vi "FrequencyAnalysis.vi"(0 "System no.":i32=1 min=1 step=1, 1 "Analog Input Channel":u32=1, 5 "error in":errorcluster) -> (19 "error out":errorcluster)   [LabVIEW 2020]
doc: "This VI allows the user to analyze oscillations on the optical path.\nFor more information, please refer to the documentation of this sample application."
uses:
  <vilib>/Utility/miscctls.llb/LVCursorListTypeDef.ctl
  C:/ProgramData/PI/LabVIEW/Low Level/GeneralCommands/Global2 (Array).vi
  <vilib>/Analysis/NI_AALPro.lvlib
panel:
  out "Sample Time":dbl format="%.10f"
  in  "Read":bool
  out "Curser X position:":dbl
  in  "Raw Data":bool
  out "2DArray":dbl[][](array[numeric])
  in  "Impulse":bool
  in  "Servo":bool=TRUE
  in  "Impulse size":dbl=1.0
  in  "Axis":u16(ring) items=["1", "2", "3", "4", "5", "6", "7", "8", "9", "10", "11", "12"]
  in  "# of data points":i32=8192
  in  "Record Rate - # cycles":i32=1
  in  "FFT":bool
  out "XY Graph":cluster{dbl[], "Data":dbl[]}(graph)
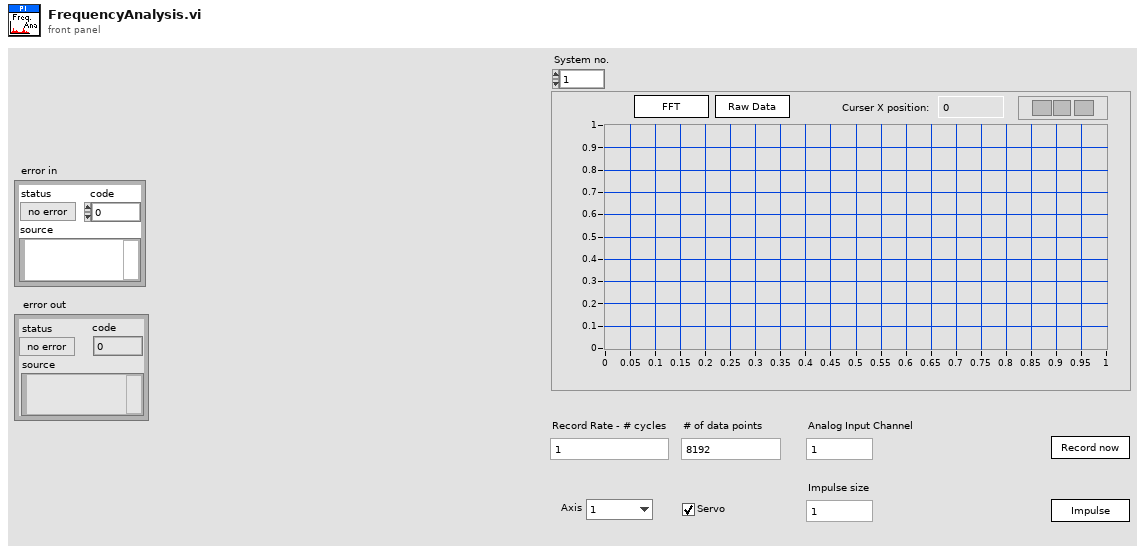
[diagram p1: front panel]
types:
  T1 = typedef "LVCursorListTypeDef.ctl" = cluster{"Name":string, "Color":u32, "Style":u8, "Point Style":u8, "Name Visible":bool, "Allow Drag":bool, "Cursor Mode":u32, "Plot":i32, "Index":i32, "Position":cluster{"X":dbl, "Y":dbl}, "X Scale":u32, "Y Scale":u32, "Watch Plots":i32[], "Watch All Plots":bool, "Plot Area":i32, "Label Offset":cluster{"X":dbl, "Y":dbl}}[]
  T2 = typedef "Controller names.ctl" = enum16{"None", "Analog", "C-702", "C-413", "C-414", "C-843", "C-843.PM", "C-844", "C-848", "C-865", "C-866", "C-867", "C-877", "C-880", "C-884", "C-885", "C-886", "C-887", "C-891", "E-135", "E-516", "E-517", "E-518", "E-709", "E-710", "E-712", "E-725", "E-727", "E-753", "E-754", "E-755", "E-761", "E-816", "E-861", "E-870", "E-871", "E-872", "E-873", "E-874", "F-206", "HydraPollux", "M-840", "M-850", "M-8X0", "Mercury", "Mercury_GCS", "PI_GCS2"}
  T3 = cluster{"Conn. axes":string[], "Controller name":T2}[]
  T4 = cluster{"Conn. axes":string[], "Controller name":T2}
  T5 = typedef "LVPoint32TypeDef.ctl" = cluster{"Horizontal":i32, "Vertical":i32}
  T6 = typedef "LVRectTypeDef.ctl" = cluster{"Left":i16, "Top":i16, "Right":i16, "Bottom":i16}
  T7 = cluster{"Name":string, "Color":u32, "Style":u8, "Point Style":u8, "Name Visible":bool, "Allow Drag":bool, "Cursor Mode":u32, "Plot":i32, "Index":i32, "Position":cluster{"X":dbl, "Y":dbl}, "X Scale":u32, "Y Scale":u32, "Watch Plots":i32[], "Watch All Plots":bool, "Plot Area":i32, "Label Offset":cluster{"X":dbl, "Y":dbl}}
  T8 = cluster{"Name":string, "Color":u32, "Style":u8, "Point Style":u8, "Name Visible":bool, "Allow Drag":bool, "Cursor Mode":u32, "Plot":i32, "Index":i32, "Position":cluster{"X":dbl, "Y":dbl}, "X Scale":u32, "Y Scale":u32, "Watch Plots":i32[], "Watch All Plots":bool, "Plot Area":i32, "Label Offset":cluster{"X":dbl, "Y":dbl}}[]
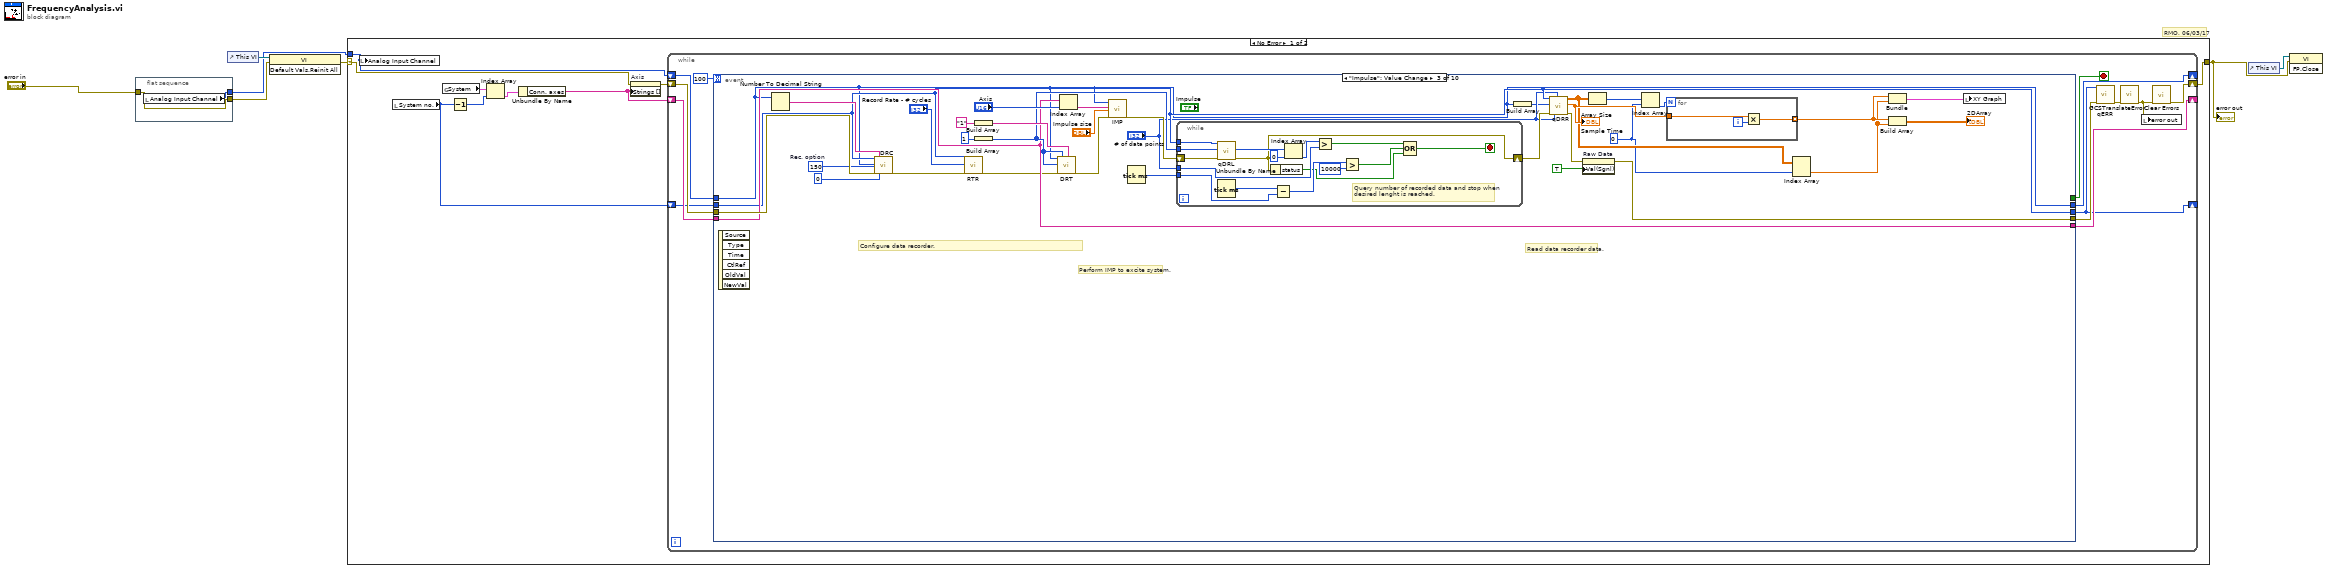
[diagram p0: block diagram]
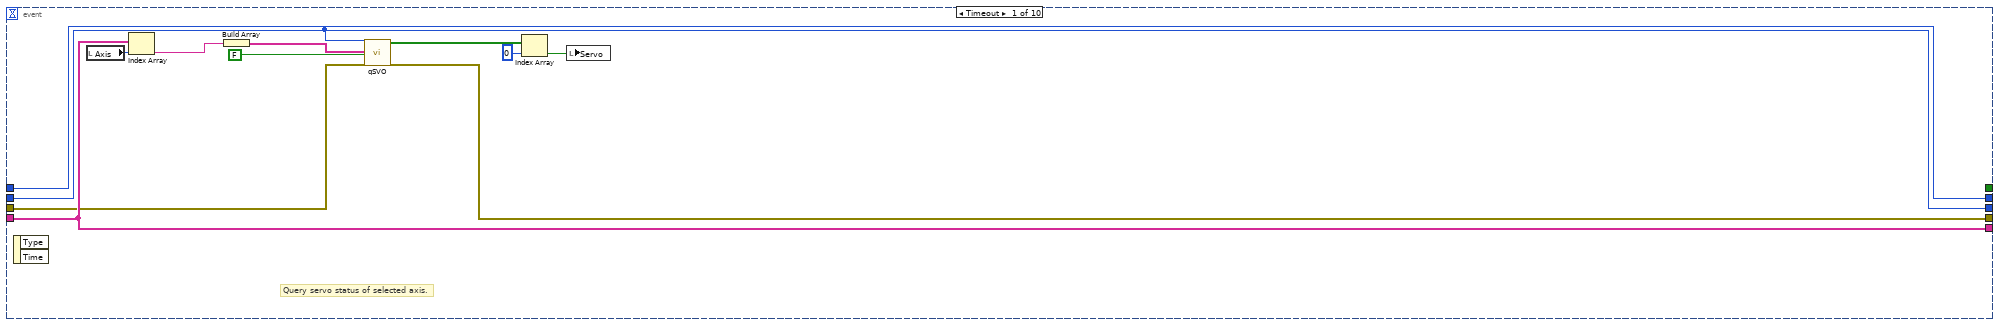
[diagram p2: hidden frame]
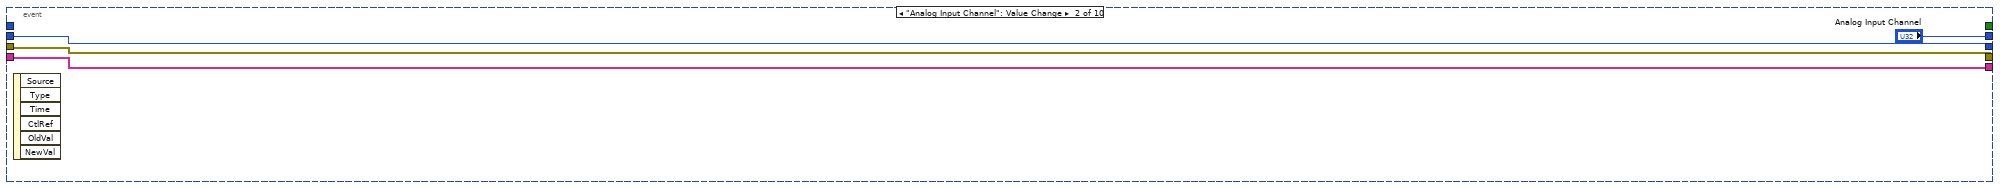
[diagram p3: hidden frame]
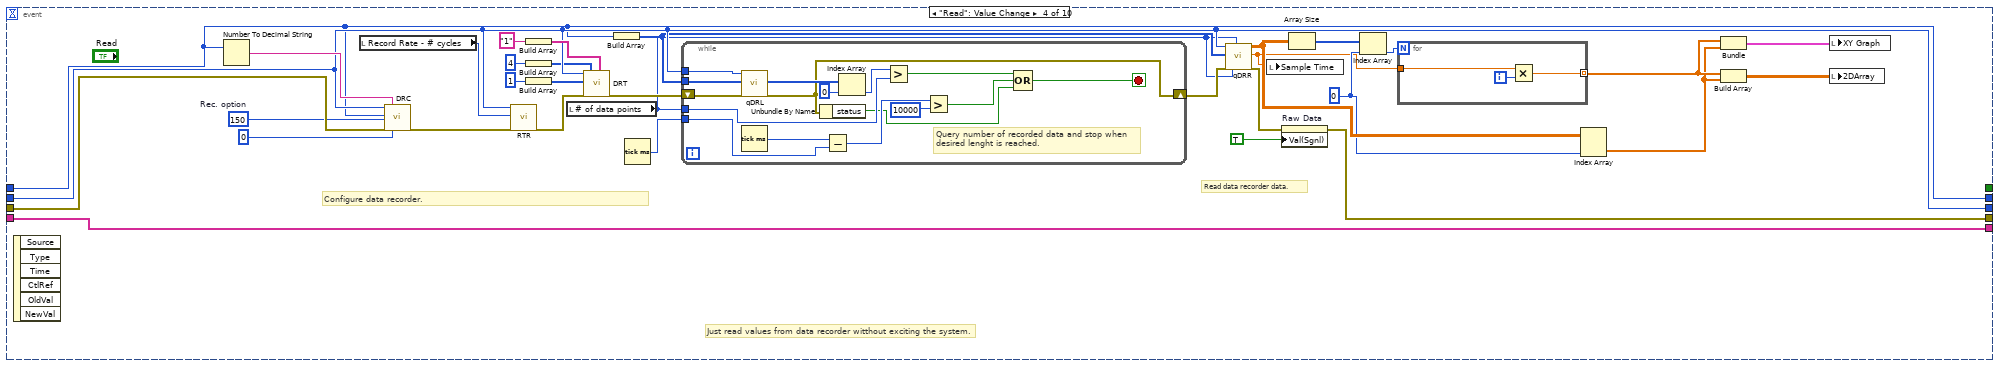
[diagram p4: hidden frame]
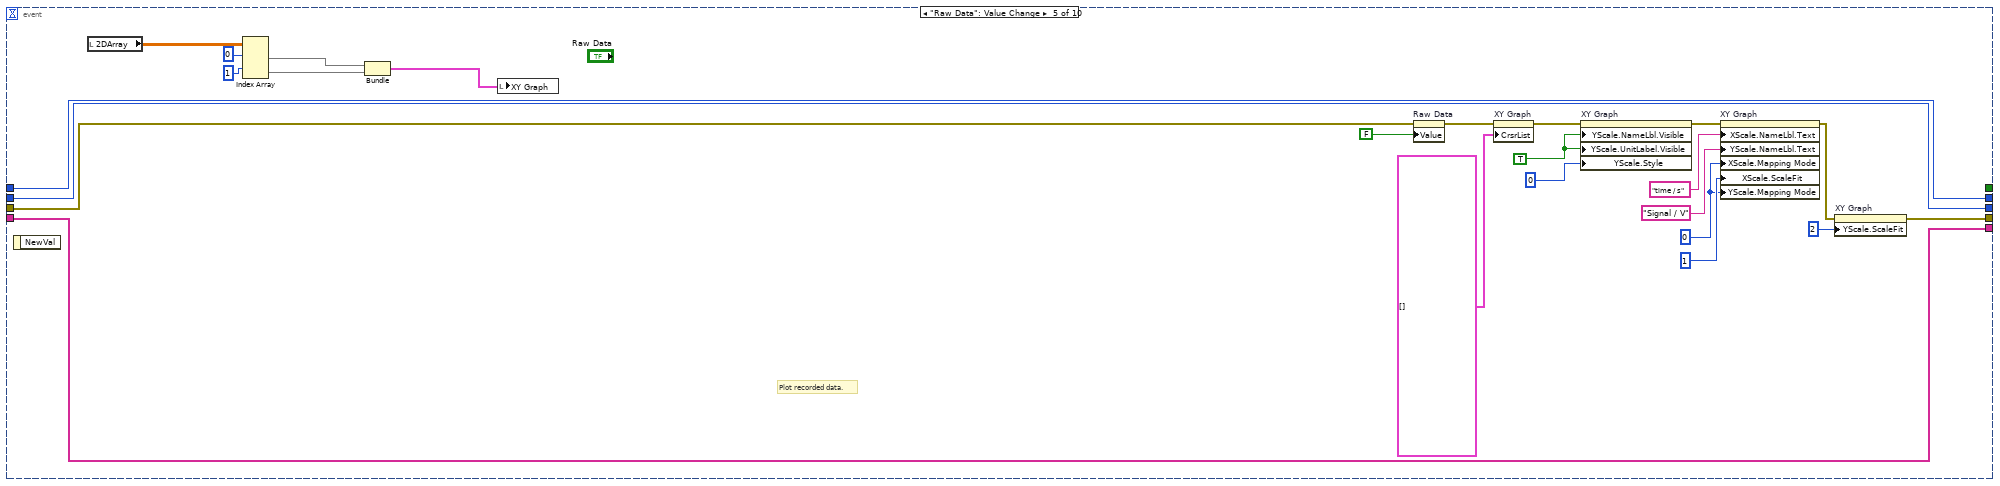
[diagram p5: hidden frame]
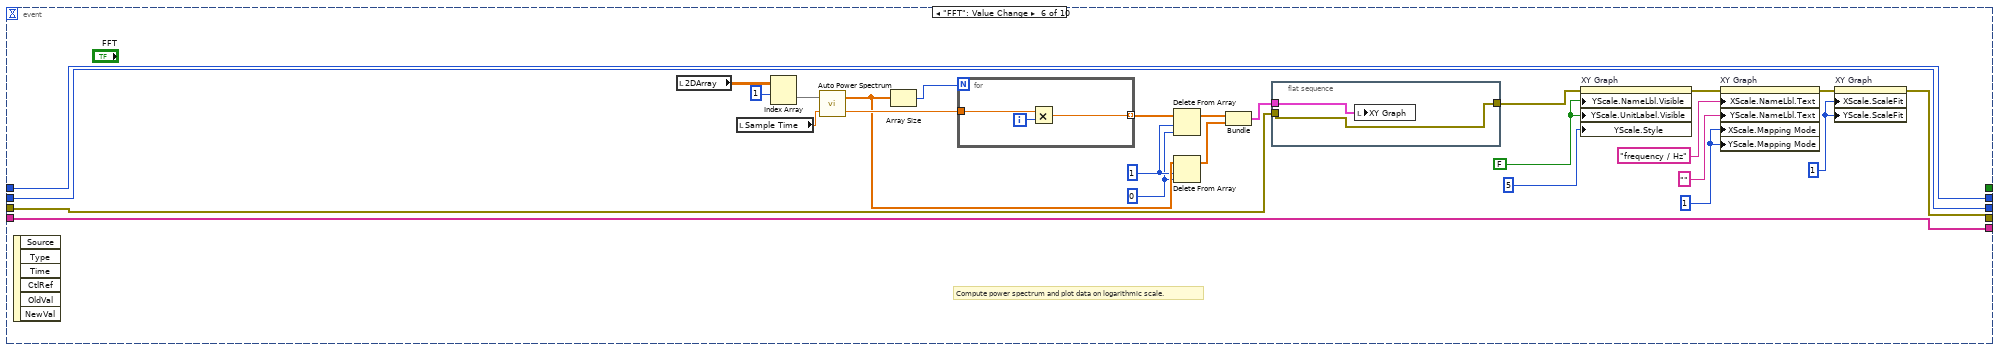
[diagram p6: hidden frame]
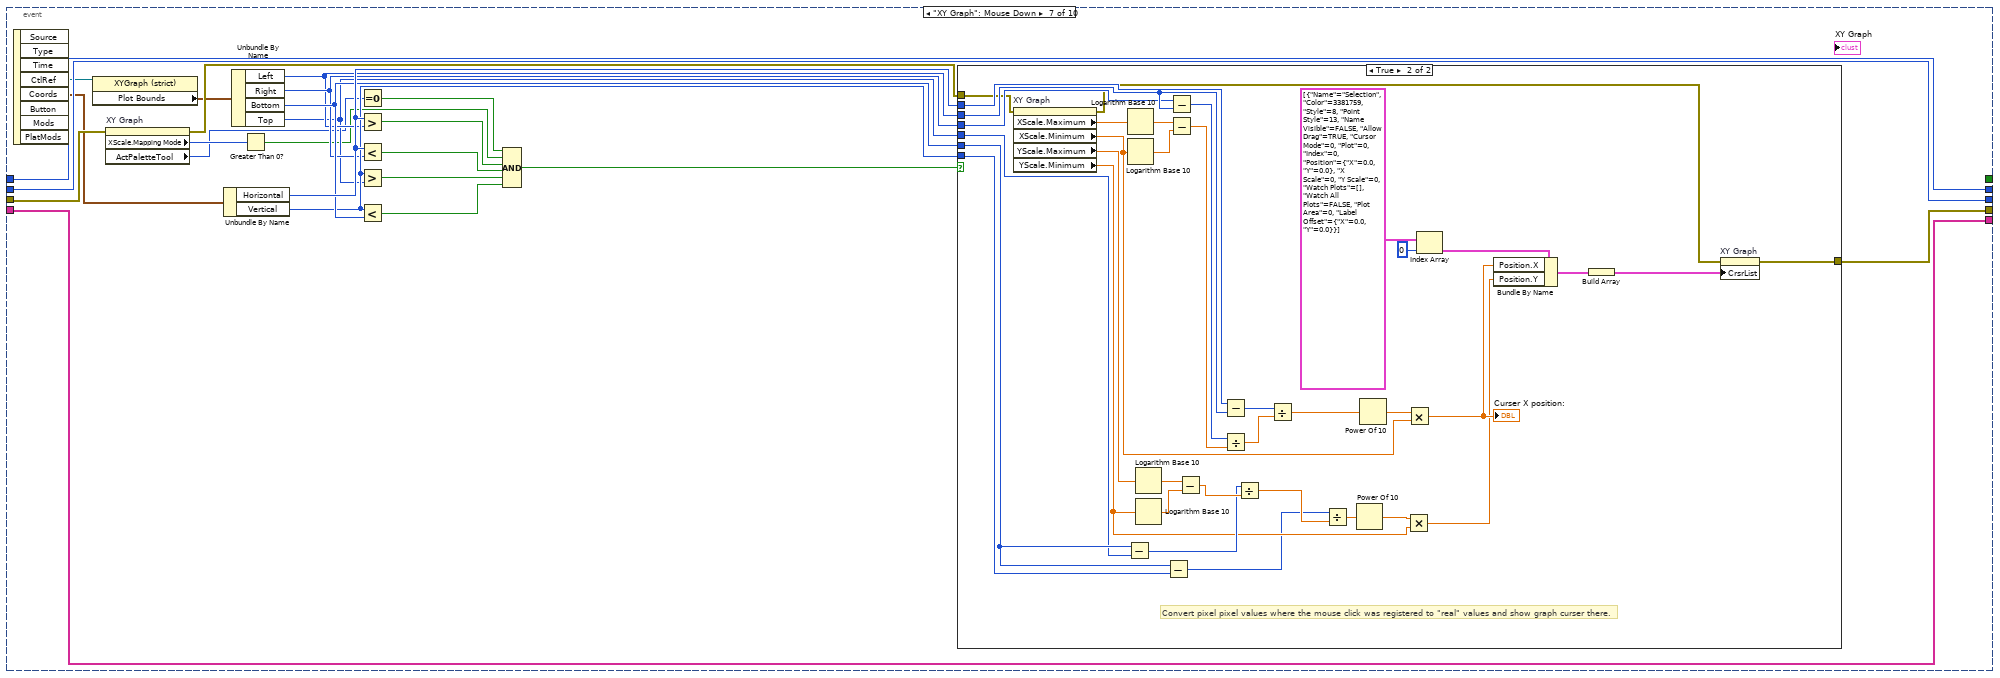
[diagram p7: hidden frame]
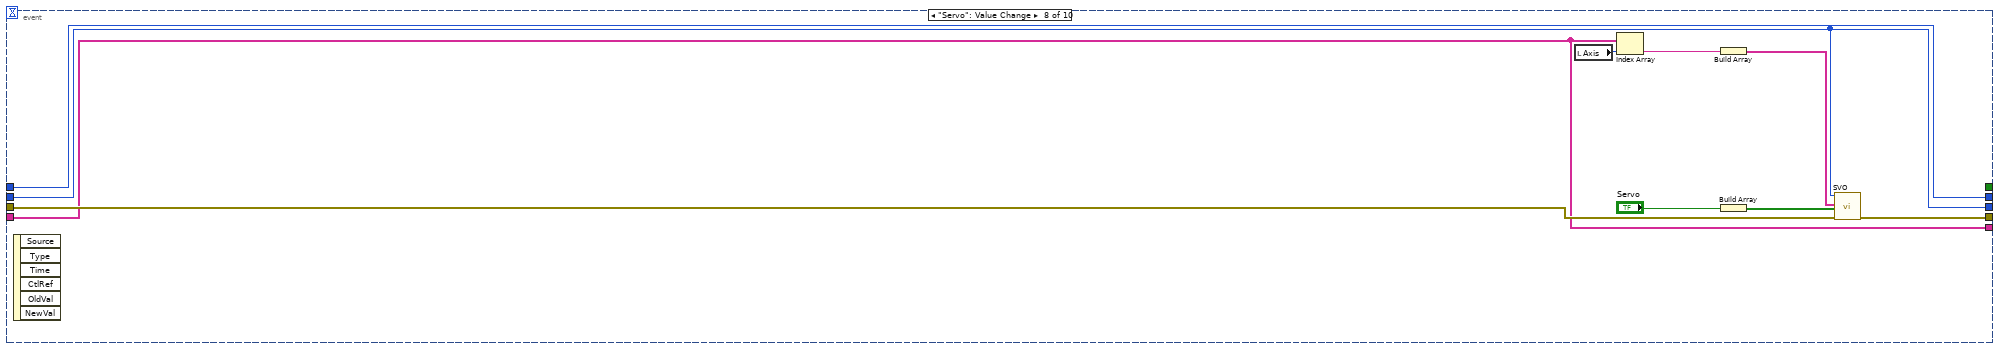
[diagram p9: hidden frame]
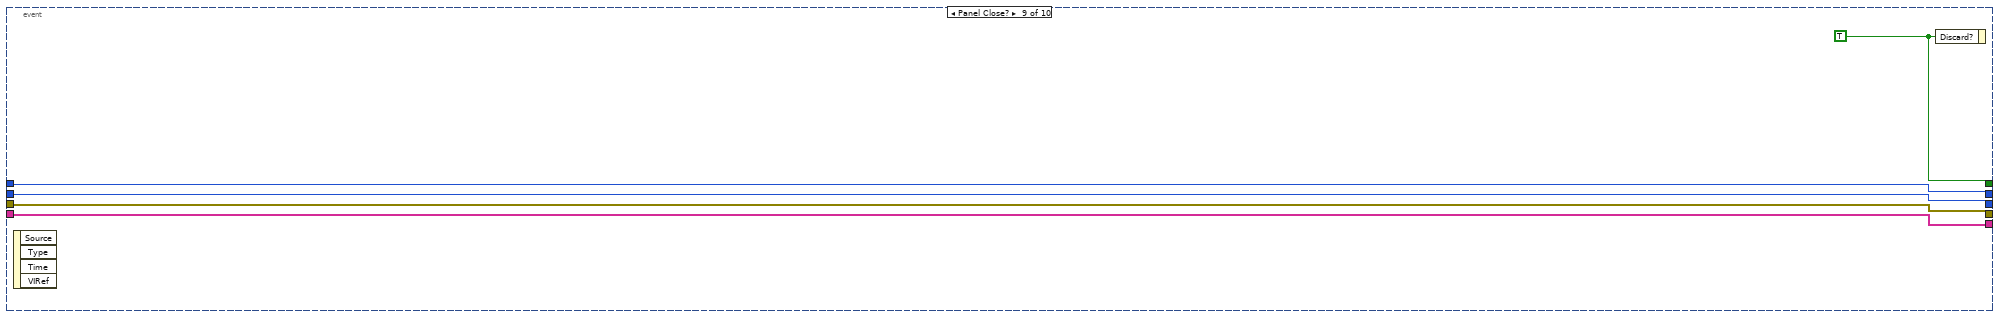
[diagram p10: hidden frame]
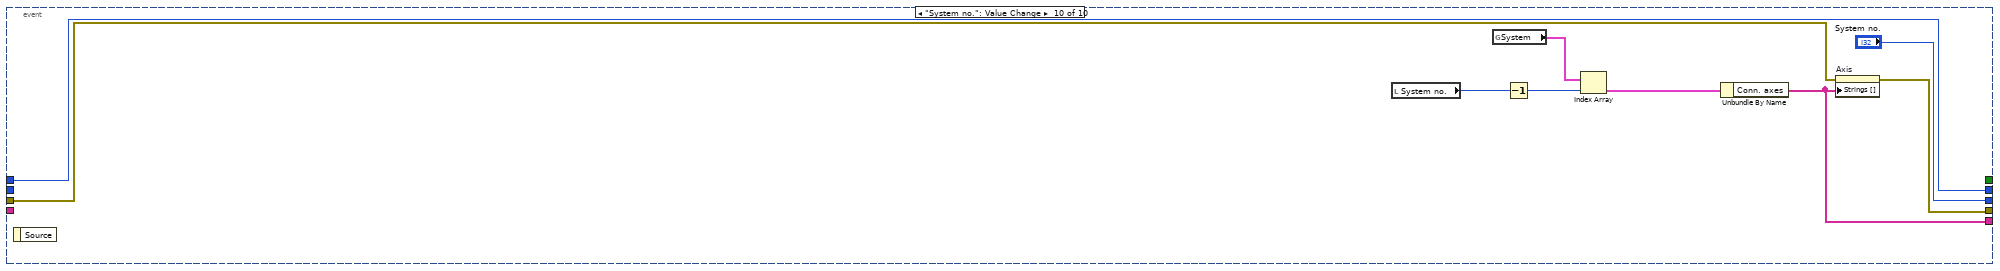
[diagram p11: hidden frame]
diagram:
  # "RMO, 06/03/17"
  n1 = flat-sequence {
    tunnel: "error in" -> [w9]
    tunnel: [w9] -> w4
    tunnel: [w8] -> w3
    frame #0 {
      n2 = local read "Analog Input Channel"() -> (w8:u32)
    }
  }
  n3 = control-ref of="This VI"() -> (w6:refnum<vi>)
  n4 = invoke class="VI" method="Default Vals.Reinit All"(reference=w6, error in=w4) -> (error out=w5:errorcluster)  [unwired: 1 in, 2 out]
  n5 = case shown="No Error" w5 {
    selector: w5 -> [w13 w295]
    tunnel: [w15 w295] -> w7
    tunnel: w3 -> [w10 _]
    frame No Error {
      n6 = local write "Analog Input Channel"(w10) -> ()
      n7 = local read "System no."() -> (w14:i32)
      n8 = global read "Global2 (Array).vi" "System"() -> (w18:T3)
      n9 = Decrement(x=w14) -> (x-1=w17:i32)
      n10 = Index Array(array=w18, index=w17) -> (element=w16:T4)
      n11 = Unbundle By Name(w16) -> ("Conn. axes"=w11:string[])
      n12 = property on="Axis" class="Ring (strict)"(error in=w13, "Strings []"=w11) -> (error out=w12:errorcluster)  [unwired: 1 in, 1 out]
      n13 = while {
        shift-right: [w24] -> w15
        shift-left: w12 -> [w30]
        shift-right: [w22] -> _
        shift-left: w11 -> [w31]
        shift-right: [w21] -> _
        shift-left: w14 -> [w25]
        shift-right: [w20] -> _
        shift-left: w10 -> [w19]
        stop <- w29 stop-if-true
        n14 = event shown="[2] \"Impulse\": Value Change" {
          selector: _ -> [_ _ _ _ _ _ _ _ _ _]
          dyn-events: _ -> [_ _ _ _ _ _ _ _ _ _]
          timeout: 100 -> [_ _ _ _ _ _ _ _ _ _]
          tunnel: w31 -> [w36 w45 w64 w122 w175 w202 w232 w274 w284 _]
          tunnel: w30 -> [w32 w44 w77 w130 w161 w183 w233 w280 w283 w290]
          tunnel: [w41 w44 w56 w115 w155 w188 w215 w273 w283 w289] -> w27
          tunnel: [_ _ _ _ _ _ _ _ w285 _] -> w29
          tunnel: w25 -> [w42 w46 w63 w121 w176 w203 w231 w272 w282 _]
          tunnel: [w36 w45 w64 w122 w175 w202 w232 w274 w284 w288] -> w22
          tunnel: [w42 w46 w63 w121 w176 w203 w231 w272 w282 "System no."] -> w21
          tunnel: [w43 "Analog Input Channel" w50 w106 w177 w204 w230 w271 w281 w287] -> w20
          tunnel: w19 -> [w43 _ w50 w106 w177 w204 w230 w271 w281 w287]
          event Timeout {
            # "Query servo status of selected axis."
            n15 = event-data() -> ()  [unwired: 3 out]
            n16 = local read "Axis"() -> (w33:u16)
            n17 = Index Array(array=w36, index=w33) -> (element=w35:string)
            n18 = Build Array(w35) -> (w34:string[])
            n19 = call "qSVO.vi"("System no."=w42, "Axes to query"=w34, "All axes?"=FALSE, "error in"=w32) -> ("Servo status?"=w40:bool[], "error out"=w41:errorcluster)  [unwired: 1 in, 13 out]
            n20 = Index Array(array=w40, index=0) -> (element=w38:bool)
            n21 = local write "Servo"(w38) -> ()
          }
          event "Analog Input Channel": Value Change {
            n22 = event-data() -> ()  [unwired: 7 out]
          }
          event "Impulse": Value Change {
            w48 = 150  # Rec. option
            w62 = 0 ("index")
            # "Read data recorder data."
            # "Perform IMP to excite system."
            # "Configure data recorder."
            n23 = event-data() -> ()  [unwired: 7 out]
            n24 = Number To Decimal String(number=w50) -> (decimal integer string=w76:string)  [unwired: 1 out]
            n25 = call "DRC.vi"("System no."=w63, "Rec. table"=w50, "Rec. option"=w48, "error in"=w77, "Source ID"=w76, "Trigger option"=0) -> ("error out"=w52:errorcluster)  [unwired: 13 out]
            n26 = call "RTR.vi"("System no."=w63, "Table rate"="Record Rate - # cycles", "error in"=w52) -> ("error out"=w53:errorcluster)  [unwired: 16 out]
            n27 = Build Array("1") -> (w80:string[])
            n28 = Build Array(1) -> (w69:i32[])
            n29 = call "DRT.vi"("System no."=w63, "DataRecorderTable"=w69, "error in"=w53, "Trigger source"=w69, "Value"=w80) -> ("error out"=w54:errorcluster)  [unwired: 14 out]
            n30 = Index Array(array=w64, index="Axis") -> (element=w74:string)
            n31 = call "IMP.vi"("System no."=w63, "Axis to command"=w74, "Impulse size"="Impulse size", "error in"=w54) -> ("error out"=w71:errorcluster)  [unwired: 1 in, 14 out]
            n32 = Tick Count (ms)() -> (millisecond timer value=w72:u32)
            n33 = while {
              tunnel: w63 -> [w101]
              tunnel: w69 -> [w100]
              tunnel: "# of data points" -> [w96]
              tunnel: w72 -> [w94]
              shift-right: [w86] -> w70
              shift-left: w71 -> [w91]
              stop <- w87 stop-if-true
              # "Query number of recorded data and stop when desired lenght is reached."
              n34 = call "qDRL.vi"("System no."=w101, "Rec. table to query"=w100, "error in"=w91) -> ("No. of rec. values"=w99:i32[], "error out"=w86:errorcluster)  [unwired: 1 in, 14 out]
              n35 = Tick Count (ms)() -> (millisecond timer value=w95:u32)
              n36 = Unbundle By Name(w86) -> ("status"=w88:bool)
              n37 = Subtract(x=w95, y=w94) -> (x-y=w93:u32)
              n38 = Index Array(array=w99, index=0) -> (element=w97:i32)
              n39 = Greater?(x=w97, y=w96) -> (0:w90:bool)
              n40 = Greater?(x=w93, y=u32 10000) -> (0:w89:bool)
              n41 = Compound Arithmetic op=OR(w90, w89, w88) -> (w87:bool)
            }
            n42 = Build Array(w50) -> (w49:u32[])
            n43 = call "qDRR.vi"("System no."=w63, "Rec. table IDs"=w49, "error in"=w70, "N"="# of data points", "Nmax"="# of data points") -> ("Data"=w65:dbl[][], "Sample Time"=w66:dbl, "error out"=w57:errorcluster)  [unwired: 3 in, 9 out]
            "Sample Time" <- w66
            n44 = property on="Raw Data" class="Bool (strict)"(error in=w57, "Val(Sgnl)"=TRUE) -> (error out=w56:errorcluster)  [unwired: 1 in, 1 out]
            n45 = Array Size(array=w65) -> (size(s)=w68:i32[])
            n46 = Index Array(array=w68, index=w62) -> (element=w67:i32)
            n47 = for {
              N: w67 -> [_]
              tunnel: w66 -> [w85]
              tunnel: [w84] -> w61 mode=indexing
              i -> [w83]
              n48 = Multiply(x=w85, y=w83) -> (x*y=w84:dbl)
            }
            n49 = Index Array(array=w65, index (col)=w62) -> (element=w60:dbl[])  [unwired: 1 in]
            n50 = Bundle(w61, "Data"=w60) -> (w58:cluster{dbl[], "Data":dbl[]})  [unwired: 1 out]
            n51 = Build Array(w61, w60) -> (→"2DArray":dbl[][])
            n52 = local write "XY Graph"(w58) -> ()
          }
          event "Read": Value Change {
            w102 = 150  # Rec. option
            w120 = 0 ("index")
            # "Just read values from data recorder witthout exciting the system."
            # "Read data recorder data."
            # "Configure data recorder."
            n53 = event-data() -> ()  [unwired: 7 out]
            n54 = Number To Decimal String(number=w106) -> (decimal integer string=w129:string)  [unwired: 1 out]
            n55 = local read "Record Rate - # cycles"() -> (w113:i32)
            n56 = call "DRC.vi"("System no."=w121, "Rec. table"=w106, "Rec. option"=w102, "error in"=w130, "Source ID"=w129, "Trigger option"=0) -> ("error out"=w109:errorcluster)  [unwired: 13 out]
            n57 = call "RTR.vi"("System no."=w121, "Table rate"=w113, "error in"=w109) -> ("error out"=w108:errorcluster)  [unwired: 16 out]
            n58 = Build Array("1") -> (w132:string[])
            n59 = Build Array(4) -> (w111:i32[])
            n60 = Build Array(1) -> (w126:i32[])
            n61 = local read "# of data points"() -> (w103:i32)
            n62 = call "DRT.vi"("System no."=w121, "DataRecorderTable"=w126, "error in"=w108, "Trigger source"=w111, "Value"=w132) -> ("error out"=w107:errorcluster)  [unwired: 14 out]
            n63 = Build Array(w106) -> (w105:u32[])
            n64 = Tick Count (ms)() -> (millisecond timer value=w128:u32)
            n65 = while {
              tunnel: w121 -> [w153]
              tunnel: w105 -> [w152]
              tunnel: w103 -> [w148]
              tunnel: w128 -> [w146]
              shift-right: [w138] -> w127
              shift-left: w107 -> [w143]
              stop <- w139 stop-if-true
              # "Query number of recorded data and stop when desired lenght is reached."
              n66 = call "qDRL.vi"("System no."=w153, "Rec. table to query"=w152, "error in"=w143) -> ("No. of rec. values"=w151:i32[], "error out"=w138:errorcluster)  [unwired: 1 in, 14 out]
              n67 = Tick Count (ms)() -> (millisecond timer value=w147:u32)
              n68 = Unbundle By Name(w138) -> ("status"=w140:bool)
              n69 = Subtract(x=w147, y=w146) -> (x-y=w145:u32)
              n70 = Index Array(array=w151, index=0) -> (element=w149:i32)
              n71 = Greater?(x=w149, y=w148) -> (0:w142:bool)
              n72 = Greater?(x=w145, y=u32 10000) -> (0:w141:bool)
              n73 = Compound Arithmetic op=OR(w142, w141, w140) -> (w139:bool)
            }
            n74 = call "qDRR.vi"("System no."=w121, "Rec. table IDs"=w105, "error in"=w127, "N"=w103, "Nmax"=w103) -> ("Data"=w123:dbl[][], "Sample Time"=w104:dbl, "error out"=w116:errorcluster)  [unwired: 3 in, 9 out]
            n75 = local write "Sample Time"(w104) -> ()
            n76 = property on="Raw Data" class="Bool (strict)"(error in=w116, "Val(Sgnl)"=TRUE) -> (error out=w115:errorcluster)  [unwired: 1 in, 1 out]
            n77 = Array Size(array=w123) -> (size(s)=w125:i32[])
            n78 = Index Array(array=w125, index=w120) -> (element=w124:i32)
            n79 = for {
              N: w124 -> [_]
              tunnel: w104 -> [w137]
              tunnel: [w136] -> w119 mode=indexing
              i -> [w135]
              n80 = Multiply(x=w137, y=w135) -> (x*y=w136:dbl)
            }
            n81 = Index Array(array=w123, index (col)=w120) -> (element=w118:dbl[])  [unwired: 1 in]
            n82 = Bundle(w119, "Data"=w118) -> (w117:cluster{dbl[], "Data":dbl[]})  [unwired: 1 out]
            n83 = Build Array(w119, w118) -> (w112:dbl[][])
            n84 = local write "XY Graph"(w117) -> ()
            n85 = local write "2DArray"(w112) -> ()
          }
          event "Raw Data": Value Change {
            w157 = u8 0 ("X Scale.Mapping Mode")
            w165 = TRUE ("Y Scale.Name Label.Visible")
            # "Plot recorded data."
            n86 = event-data() -> ()  [unwired: 2 out]
            n87 = local read "2DArray"() -> (w172:dbl[][])
            n88 = Index Array(array=w172, index (row) #1=0 ("disabled index (col)"), index (row) #2=1 ("disabled index (col)")) -> (element #1=w171:dbl[], element #2=w170:dbl[])  [unwired: 2 in]
            n89 = Bundle("2DArray"=w171, "2DArray"=w170) -> (w169:cluster{"2DArray":dbl[], "2DArray":dbl[]})  [unwired: 1 out]
            n90 = local write "XY Graph"(w169) -> ()
            n91 = property on="Raw Data" class="Bool (strict)"(error in=w161, "Value"=FALSE) -> (error out=w160:errorcluster)  [unwired: 1 in, 1 out]
            n92 = property on="XY Graph" class="XYGraph (strict)"(error in=w160, "CrsrList"=T1 [] ("Cursor List")) -> (error out=w163:errorcluster)  [unwired: 1 in, 1 out]
            n93 = property on="XY Graph" class="XYGraph (strict)"(error in=w163, "YScale.NameLbl.Visible"=w165, "YScale.UnitLabel.Visible"=w165, "YScale.Style"=u8 0 ("Y Scale.Style")) -> (error out=w166:errorcluster)  [unwired: 1 in, 1 out]
            n94 = property on="XY Graph" class="XYGraph (strict)"(error in=w166, "XScale.NameLbl.Text"="time / s" ("X Scale.Name Label.Text"), "YScale.NameLbl.Text"="Signal / V" ("Y Scale.Name Label.Text"), "XScale.Mapping Mode"=w157, "XScale.ScaleFit"=1, "YScale.Mapping Mode"=w157) -> (error out=w156:errorcluster)  [unwired: 1 in, 1 out]
            n95 = property on="XY Graph" class="XYGraph (strict)"(error in=w156, "YScale.ScaleFit"=2) -> (error out=w155:errorcluster)  [unwired: 1 in, 1 out]
          }
          event "FFT": Value Change {
            w180 = u8 1 ("X Scale.Scale Fit")
            w181 = u8 1 ("X Scale.Mapping Mode")
            w186 = FALSE
            w194 = 0 ("index")
            w195 = 1 ("index")
            # "Compute power spectrum and plot data on logarithmic scale."
            n96 = event-data() -> ()  [unwired: 7 out]
            n97 = local read "2DArray"() -> (w178:dbl[][])
            n98 = local read "Sample Time"() -> (w184:dbl)
            n99 = Index Array(array=w178, index (row)=1 ("disabled index (col)")) -> (element=w179:dbl[])  [unwired: 1 in]
            n100 = call <vilib>:"Auto Power Spectrum.vi"("dt"=w184, "Signal (V)"=w179) -> ("df"=w200:dbl, "Power Spectrum (V^2 rms)"=w197:dbl[])
            n101 = Array Size(array=w197) -> (size(s)=w199:i32)
            n102 = for {
              N: w199 -> [_]
              tunnel: w200 -> [w209]
              tunnel: [w208] -> w196 mode=indexing
              i -> [w207]
              n103 = Multiply(x=w209, y=w207) -> (x*y=w208:dbl)
            }
            n104 = Delete From Array(array=w196, length=w195, index=w194) -> (array with subset deleted=w193:dbl[])  [unwired: 1 out]
            n105 = Delete From Array(array=w197, length=w195, index=w194) -> (array with subset deleted=w192:dbl[])  [unwired: 1 out]
            n106 = Bundle(w193, "Power Spectrum (V^2 rms)"=w192) -> (w198:cluster{dbl[], "Power Spectrum (V^2 rms)":dbl[]})  [unwired: 1 out]
            n107 = flat-sequence {
              tunnel: w198 -> [w206]
              tunnel: w183 -> [w205]
              tunnel: [w205] -> w182
              frame #0 {
                n108 = local write "XY Graph"(w206) -> ()
              }
            }
            n109 = property on="XY Graph" class="XYGraph (strict)"(error in=w182, "YScale.NameLbl.Visible"=w186, "YScale.UnitLabel.Visible"=w186, "YScale.Style"=u8 5 ("Y Scale.Style")) -> (error out=w187:errorcluster)  [unwired: 1 in, 1 out]
            n110 = property on="XY Graph" class="XYGraph (strict)"(error in=w187, "XScale.NameLbl.Text"="frequency / Hz" ("X Scale.Name Label.Text"), "YScale.NameLbl.Text"="" ("Y Scale.Name Label.Text"), "XScale.Mapping Mode"=w181, "YScale.Mapping Mode"=w181) -> (error out=w189:errorcluster)  [unwired: 1 in, 1 out]
            n111 = property on="XY Graph" class="XYGraph (strict)"(error in=w189, "XScale.ScaleFit"=w180, "YScale.ScaleFit"=w180) -> (error out=w188:errorcluster)  [unwired: 1 in, 1 out]
          }
          event "XY Graph": Mouse Down {
            n112 = event-data() -> ("CtlRef"=w228:refnum<vi>, "Coords"=w222:T5)  [unwired: 7 out]
            n113 = property class="XYGraph (strict)"(reference=w228) -> ("Plot Bounds"=w227:T6)  [unwired: 1 in, 2 out]
            n114 = property on="XY Graph" class="XYGraph (strict)"(error in=w233) -> (error out=w229:errorcluster, "XScale.Mapping Mode"=w213:u8, "ActPaletteTool"=w211:i32)  [unwired: 1 in, 1 out]
            n115 = Unbundle By Name(w222) -> ("Horizontal"=w221:i32, "Vertical"=w219:i32)
            n116 = Unbundle By Name(w227) -> ("Left"=w217:i16, "Right"=w218:i16, "Bottom"=w220:i16, "Top"=w216:i16)
            n117 = Greater Than 0?(x=w213) -> (x > 0?=w212:bool)
            n118 = Equal To 0?(x=w211) -> (x = 0?=w210:bool)
            n119 = Greater?(x=w221, y=w217) -> (0:w226:bool)
            n120 = Less?(x=w221, y=w218) -> (x < y?=w225:bool)
            n121 = Greater?(x=w219, y=w216) -> (0:w224:bool)
            n122 = Less?(x=w219, y=w220) -> (x < y?=w223:bool)
            n123 = Compound Arithmetic op=AND(w210, w212, w226, w225, w224, w223) -> (w214:bool)
            n124 = case shown="True" w214 {
              tunnel: w229 -> [w234 w259]
              tunnel: [w234 w270] -> w215
              tunnel: w218 -> [_ w260]
              tunnel: w221 -> [_ w262]
              tunnel: w220 -> [_ w264]
              tunnel: w219 -> [_ w265]
              tunnel: w217 -> [_ w261]
              tunnel: w216 -> [_ w263]
              frame False {
              }
              frame True {
                # "Convert pixel pixel values where the mouse click was registered to \"real\" values and show graph curser there."
                n125 = property on="XY Graph" class="XYGraph (strict)"(error in=w259) -> (error out=w258:errorcluster, "XScale.Maximum"=w257:dbl, "XScale.Minimum"=w248:dbl, "YScale.Maximum"=w244:dbl, "YScale.Minimum"=w238:dbl)  [unwired: 1 in, 1 out]
                n126 = Subtract(x=w264, y=w263) -> (x-y=w241:i16)
                n127 = Logarithm Base 10(1:w257) -> (0:w256:dbl)
                n128 = Logarithm Base 10(1:w248) -> (0:w245:dbl)
                n129 = Logarithm Base 10(1:w244) -> (0:w246:dbl)
                n130 = Logarithm Base 10(1:w238) -> (0:w247:dbl)
                n131 = Subtract(x=w264, y=w265) -> (x-y=w236:i32)
                n132 = Subtract(x=w260, y=w261) -> (x-y=w255:i16)
                n133 = Subtract(x=w256, y=w245) -> (x-y=w254:dbl)
                n134 = Subtract(x=w246, y=w247) -> (x-y=w243:dbl)
                n135 = Subtract(x=w262, y=w261) -> (x-y=w252:i32)
                n136 = Divide(x=w255, y=w254) -> (x/y=w253:dbl)
                n137 = Divide(x=w241, y=w243) -> (x/y=w242:dbl)
                n138 = Divide(x=w252, y=w253) -> (x/y=w251:dbl)
                n139 = Divide(x=w236, y=w242) -> (x/y=w240:dbl)
                n140 = Power Of 10(x=w240) -> (10^x=w239:dbl)
                n141 = Power Of 10(x=w251) -> (10^x=w250:dbl)
                n142 = Multiply(x=w239, y=w238) -> (x*y=w237:dbl)
                n143 = Multiply(x=w250, y=w248) -> (x*y=w249:dbl)
                "Curser X position:" <- w249
                n144 = Index Array(array=T1 [{"Name"="Selection", "Color"=3381759, "Style"=8, "Point Style"=13, "Name Visible"=FALSE, "Allow Drag"=TRUE, "Cursor Mode"=0, "Plot"=0, "Index"=0, "Position"={"X"=0.0, "Y"=0.0}, "X Scale"=0, "Y Scale"=0, "Watch Plots"=[], "Watch All Plots"=FALSE, "Plot Area"=0, "Label Offset"={"X"=0.0, "Y"=0.0}}] ("Cursor List"), index=0) -> (element=w268:T7)
                n145 = Bundle By Name(cluster=w268, "Position.X"=w249, "Position.Y"=w237) -> (w267:T7)
                n146 = Build Array(w267) -> (w235:T8)
                n147 = property on="XY Graph" class="XYGraph (strict)"(error in=w258, "CrsrList"=w235) -> (error out=w270:errorcluster)  [unwired: 1 in, 1 out]
              }
            }
          }
          event "Servo": Value Change {
            n148 = event-data() -> ()  [unwired: 7 out]
            n149 = local read "Axis"() -> (w279:u16)
            n150 = Index Array(array=w274, index=w279) -> (element=w278:string)
            n151 = Build Array(w278) -> (w275:string[])
            n152 = Build Array("Servo") -> (w276:bool[])
            n153 = call "SVO.vi"("System no."=w272, "Axes to command"=w275, "Servo mode"=w276, "error in"=w280) -> ("error out"=w273:errorcluster)  [unwired: 1 in, 14 out]
          }
          event Panel Close? {
            w285 = TRUE
            n154 = event-data() -> ()  [unwired: 5 out]
            n155 = event-data("Discard?"=w285) -> ()  [unwired: 1 in, 1 out]
          }
          event "System no.": Value Change {
            n156 = event-data() -> ()  [unwired: 2 out]
            n157 = local read "System no."() -> (w286:i32)
            n158 = global read "Global2 (Array).vi" "System"() -> (w292:T3)
            n159 = Decrement(x=w286) -> (x-1=w293:i32)
            n160 = Index Array(array=w292, index=w293) -> (element=w294:T4)
            n161 = Unbundle By Name(w294) -> ("Conn. axes"=w288:string[])
            n162 = property on="Axis" class="Ring (strict)"(error in=w290, "Strings []"=w288) -> (error out=w289:errorcluster)  [unwired: 1 in, 1 out]
          }
        }
        n163 = call "qERR.vi"("System no."=w21, "error in"=w27) -> ("error out"=w26:errorcluster)  [unwired: 17 out]
        n164 = call "GCSTranslateError.vi"("error in"=w26) -> ("error out"=w23:errorcluster)  [unwired: 18 out]
        n165 = local write "error out"(w23) -> ()
        n166 = call <vilib>:"Clear Errors.vi"("error in (no error)"=w23) -> ("error out"=w24:errorcluster)  [unwired: 1 in, 5 out]
      }
    }
    frame Error {
    }
  }
  "error out" <- w7
  n167 = control-ref of="This VI"() -> (w2:refnum<vi>)
  n168 = invoke class="VI" method="FP.Close"(reference=w2, error in=w7) -> ()  [unwired: 1 in, 3 out]
